vi "db_.vi"(7 "DB File":path=path "D:/Valeo/Micriphone Test/UI/data.s3db", 8 "error in (no error)":errorcluster, 10 "Datas In":dbl[](array[numeric]), 11 "Model":string="ME79") -> (0 "error out":errorcluster, 1 "SN":string, 2 "Last INSERT RowID":i64)   [LabVIEW 2018]
uses:
  <vilib>/drjdpowell/SQLite Library/SQL Connection/Connection.lvclass/Connection.ctl
  <vilib>/drjdpowell/SQLite Library/SQL Connection/Open (path).vi
  <vilib>/drjdpowell/SQLite Library/SQL Connection/Open (string).vi
  <vilib>/AdvancedString/Path To Command Line String.vi
  <vilib>/drjdpowell/SQLite Library/SQL Connection/Execute SQL (Single Integer).vi
  <vilib>/drjdpowell/SQLite Library/SQL Connection/Execute SQL (No results).vi
  <vilib>/drjdpowell/SQLite Library/SQL Connection/Connection.lvclass
  <vilib>/drjdpowell/SQLite Library/SQLite.lvlib
panel:
  out "date/time string":string
  out "sql":string
  out "Model Id":i64
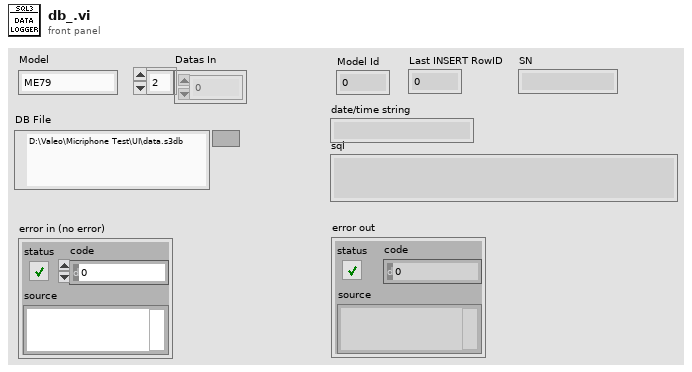
[diagram p1: front panel]
types:
  T1 = enum16{"New or existing", "Existing", "Read only"}
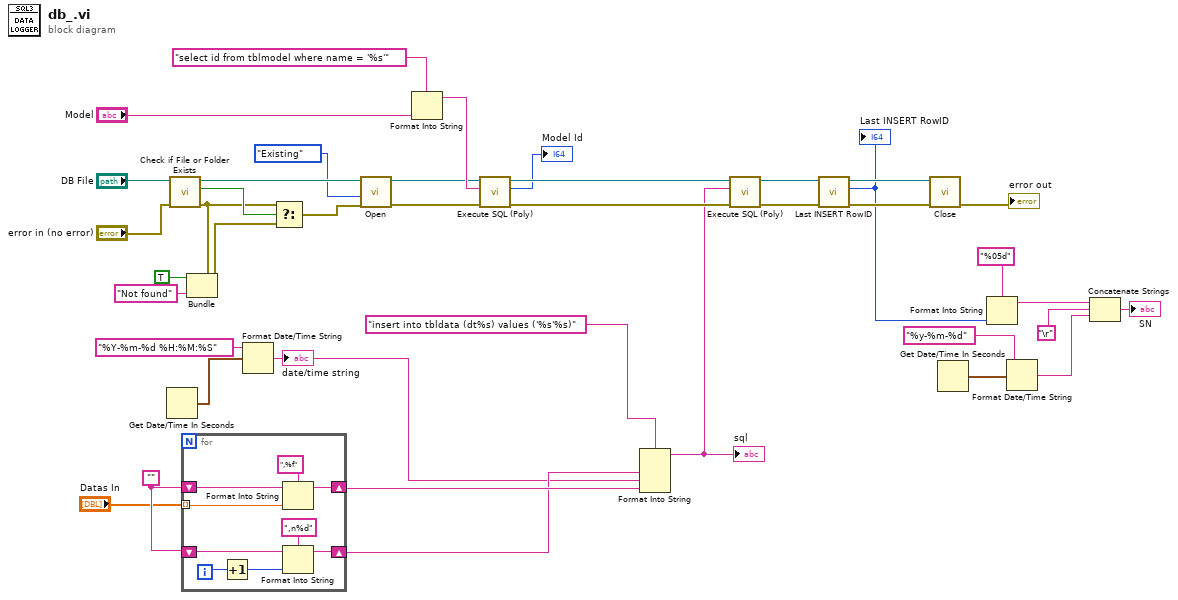
[diagram p0: block diagram]
diagram:
  w21 = ""
  n1 = Get Date/Time In Seconds() -> (seconds since 1Jan1904=w19:timestamp)
  n2 = call <vilib>:"Check if File or Folder Exists.vi"("error in (no error)"="error in (no error)", "path"="DB File") -> ("error out"=w35:errorcluster, "file or folder exists?"=w36:bool, "dup path"=w33:path)  [unwired: 7 in]
  n3 = for {
    tunnel: "Datas In" -> [w49] mode=indexing
    shift-right: [w44] -> w25
    shift-left: w21 -> [w41]
    shift-right: [w43] -> w24
    shift-left: w21 -> [w42]
    i -> [w48]
    n4 = Increment(x=w48) -> (x+1=w47:i32)
    n5 = Format Into String(format string=",%f", initial string=w41, w49) -> (resulting string=w44:string)  [unwired: 1 in, 1 out]
    n6 = Format Into String(format string=",n%d", initial string=w42, w47) -> (resulting string=w43:string)  [unwired: 1 in, 1 out]
  }
  n7 = Bundle(cluster=w35, "status"=TRUE, "source"="Not found") -> (w34:errorcluster)  [unwired: 1 in]
  n8 = Format Date/Time String(time format string (%c)="%Y-%m-%d %H:%M:%S", seconds (now)=w19) -> (date/time string=w23:string)  [unwired: 1 in]
  "date/time string" <- w23
  n9 = Select(t=w35, s=w36, f=w34) -> (s? t:f=w31:errorcluster)
  n10 = call-poly <vilib>:"Open.vi"("error in (no error)"=w31, "File Option"=T1."Existing", "db file"=w33) -> ("error out"=w28:errorcluster, "SQLite Connection"=w27:refnum<class "Connection.lvclass">)  [unwired: 7 in]
  n11 = Format Into String(format string="select id from tblmodel where name = '%s'", "Model") -> (resulting string=w29:string)  [unwired: 2 in, 1 out]
  n12 = call-poly <vilib>:"Execute SQL (Poly).vi"("error in (no error)"=w28, "SQL"=w29, "SQLite Connection in"=w27) -> ("error out"=w16:errorcluster, "Result"=→"Model Id":i64, "SQLite Connection"=w17:refnum<class "Connection.lvclass">)  [unwired: 6 in]
  n13 = Format Into String(format string="insert into tbldata (dt%s) values ('%s'%s)", w24, w23, w25) -> (resulting string=w15:string)  [unwired: 2 in, 1 out]
  "sql" <- w15
  n14 = call-poly <vilib>:"Execute SQL (Poly).vi"("error in (no error)"=w16, "SQL"=w15, "SQLite Connection in"=w17) -> ("error out"=w11:errorcluster, "SQLite Connection"=w12:refnum<class "Connection.lvclass">)  [unwired: 7 in]
  n15 = call <vilib>:"Last INSERT RowID.vi"("error in (no error)"=w11, "SQLite Connection in"=w12) -> ("error out"=w10:errorcluster, "Last INSERT RowID"=w6:i64, "SQLite Connection"=w9:refnum<class "Connection.lvclass">)  [unwired: 7 in]
  "Last INSERT RowID" <- w6
  n16 = call-dynamic "Close.vi"("error in (no error)"=w10, "SQLite Connection in"=w9) -> ("error out"=→"error out":errorcluster)  [unwired: 9 in]
  n17 = Get Date/Time In Seconds() -> (seconds since 1Jan1904=w7:timestamp)
  n18 = Format Into String(format string="%05d", w6) -> (resulting string=w4:string)  [unwired: 2 in, 1 out]
  n19 = Format Date/Time String(time format string (%c)="%y-%m-%d", seconds (now)=w7) -> (date/time string=w2:string)  [unwired: 1 in]
  n20 = Concatenate Strings(w4, "\r", w2) -> (→"SN":string)
